vi "ZLIB Specific Path to Common Path.vi"(10 "specific path":path) -> (2 "common path":string)   [LabVIEW 2022 SP3]
panel:
  out "error out":errorcluster
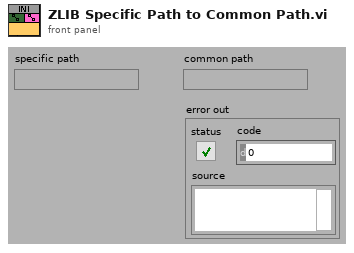
[diagram p1: front panel]
types:
  T1 = enum32{"invalid OS target", "Mac OS", "Windows 3.1", "Windows 95/NT", "Solaris 1", "Solaris 2", "HP-UX", "PowerMAX", "Linux", "Irix", "Rhapsody", "BeOS", "AIX", "OSF1", "VxWorks", "PharLap", "Carbon", "RTX", "Windows x64", "Linux x64", "Mac OS X x64"}
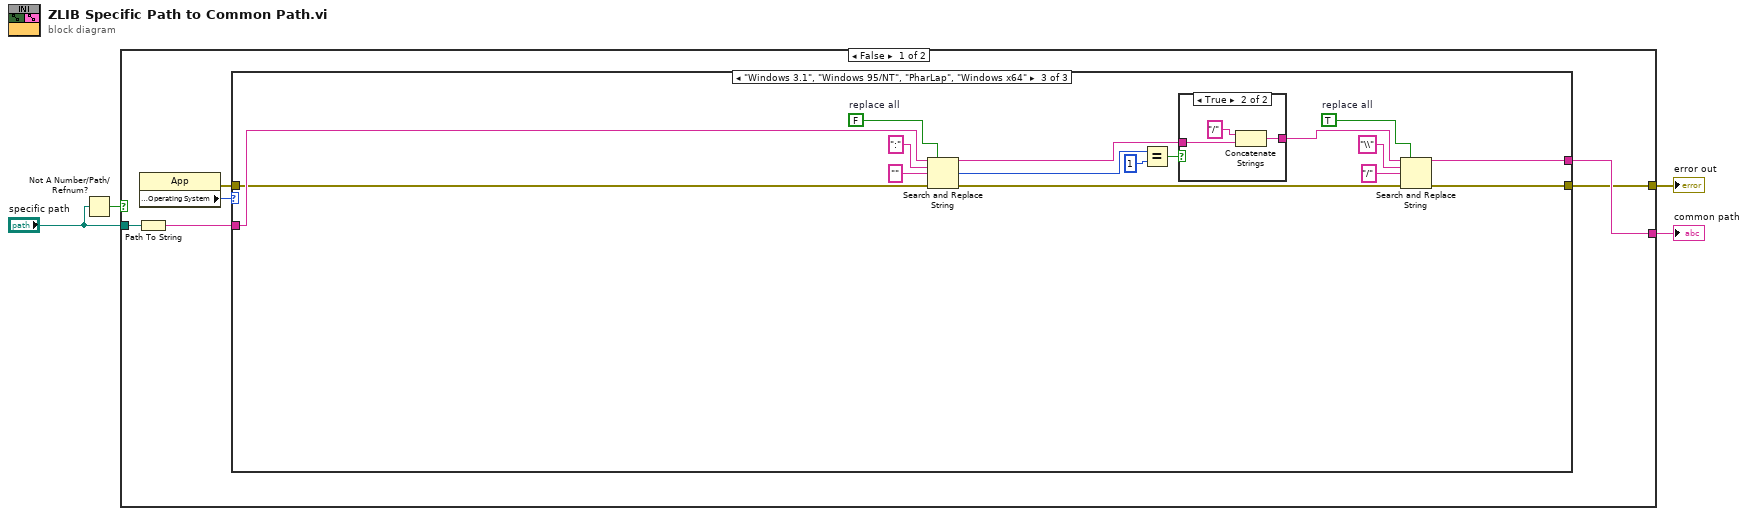
[diagram p0: block diagram]
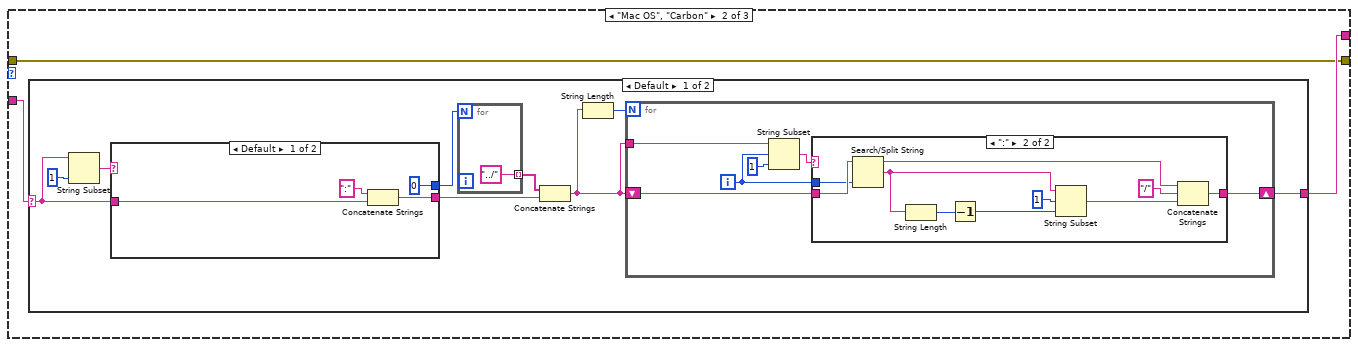
[diagram p3: hidden frame]
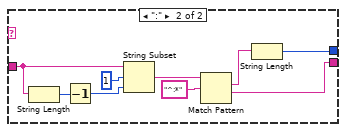
[diagram p5: hidden frame]
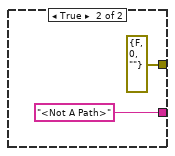
[diagram p8: hidden frame]
diagram:
  n1 = Not A Number/Path/Refnum?(number/path/refnum="specific path") -> (NaN/Path/Refnum?=w4:bool)
  n2 = case shown="False" w4 {
    tunnel: "specific path" -> [w10 _]
    tunnel: [w8 "<Not A Path>" ("string")] -> w2
    tunnel: [w5 errorcluster {"status"=FALSE, "code"=0, "source"=""} ("error out")] -> w1
    frame False {
      n3 = Path To String(path=w10) -> (string=w9:string)
      n4 = property class="App"() -> (error out=w6:errorcluster, "Application:Target:Operating System"=w7:T1)  [unwired: 2 in, 1 out]
      n5 = case shown="\"Windows 3.1\", \"Windows 95/NT\", \"PharLap\", \"Windows x64\"" w7 {
        tunnel: w9 -> [w12 w15 w67]
        tunnel: [w12 w14 w68] -> w8
        tunnel: w6 -> [w11 w13 w64]
        tunnel: [w11 w13 w69] -> w5
        frame "Linux", "VxWorks", Default {
        }
        frame "Mac OS", "Carbon" {
          n6 = case shown="Default" w15 {
            selector: w15 -> [w17 w56]
            tunnel: [w18 w56] -> w14
            frame Default {
              n7 = String Subset(string=w17, length (rest)=1 ("length")) -> (substring=w16:string)  [unwired: 1 out]
              n8 = case shown="Default" w16 {
                tunnel: w17 -> [w46 w47]
                tunnel: [w44 w50] -> w22
                tunnel: [0 w49] -> w23
                frame Default {
                  n9 = Concatenate Strings(":", w46) -> (w44:string)
                }
                frame ":" {
                  n10 = String Length(string=w47) -> (length=w55:i32)
                  n11 = Decrement(x=w55) -> (x-1=w54:i32)
                  n12 = String Subset(string=w47, offset (0)=1 ("length"), length (rest)=w54) -> (substring=w48:string)
                  n13 = Match Pattern(string=w48, regular expression="^:*") -> (match substring=w51:string, after substring=w50:string)  [unwired: 3 out]
                  n14 = String Length(string=w51) -> (length=w49:i32)
                }
              }
              n15 = for {
                N: w23 -> [_]
                tunnel: ["../"] -> w21 mode=indexing
              }
              n16 = Concatenate Strings(w21, w22) -> (w19:string)
              n17 = String Length(string=w19) -> (length=w20:i32)
              n18 = for {
                N: w20 -> [_]
                tunnel: w19 -> [w28]
                shift-right: [w29] -> w18
                shift-left: w19 -> [w30]
                i -> [w27]
                n19 = String Subset(string=w28, offset (0)=w27, length (rest)=1 ("length")) -> (substring=w25:string)
                n20 = case shown="\":\"" w25 {
                  tunnel: w30 -> [w31 w41]
                  tunnel: w27 -> [_ w33]
                  tunnel: [w31 w39] -> w29
                  frame Default {
                  }
                  frame ":" {
                    n21 = Search/Split String(string=w41, offset (0)=w33) -> (substring before match=w40:string, match + rest of string=w37:string)  [unwired: 2 out]
                    n22 = String Length(string=w37) -> (length=w36:i32)
                    n23 = Decrement(x=w36) -> (x-1=w35:i32)
                    n24 = String Subset(string=w37, offset (0)=1, length (rest)=w35) -> (substring=w32:string)
                    n25 = Concatenate Strings(w40, "/" ("x"), w32) -> (w39:string)
                  }
                }
              }
            }
            frame "" {
            }
          }
        }
        frame "Windows 3.1", "Windows 95/NT", "PharLap", "Windows x64" {
          w62 = FALSE  # replace all
          w70 = TRUE  # replace all
          n26 = Search and Replace String(replace all?=w62, input string=w67, search string=":" ("search string/char (-)"), replace string="" ("replace string (\"\")"), error in=w64) -> (result string=w58:string, number of replacements=w61:i32, error out=w63:errorcluster)  [unwired: 3 in, 1 out]
          n27 = Equal?(x=w61, y=1) -> (x = y?=w59:bool)
          n28 = case shown="True" w59 {
            tunnel: [w73 w75] -> w57
            tunnel: w58 -> [w73 w76]
            frame False {
            }
            frame True {
              n29 = Concatenate Strings("/" ("string"), w76) -> (w75:string)
            }
          }
          n30 = Search and Replace String(replace all?=w70, input string=w57, search string="\\", replace string="/" ("replace string (\"\")"), error in=w63) -> (result string=w68:string, error out=w69:errorcluster)  [unwired: 3 in, 2 out]
        }
      }
    }
    frame True {
    }
  }
  "common path" <- w2
  "error out" <- w1
